vi "Set 2D Field (Polar)_mb.vi"(5 "error in":T2, 6 "f (radians)":dbl min=0.0 format="%.3f", 8 "Z-Axis Communications Config":T1={"GPIB address"=22, "GPIB bus"=0, "connection ID"=refnum, "IP"="192.168.2.200", "Active Comm Interface"=0, "Serial Port"="", "Programmer Type"=0} {"Programmer Type" items=["Model 430", "Model 420"]; "Active Comm Interface" items=["TCP/IP (Model 430 Only)", "RS232", "IEEE488"]}, 9 "Magnitude Limit (kG)":dbl format="%.3f", 10 "Y-Axis Communications Config":T1={"GPIB address"=22, "GPIB bus"=0, "connection ID"=refnum, "IP"="192.168.2.200", "Active Comm Interface"=0, "Serial Port"="", "Programmer Type"=0} {"Programmer Type" items=["Model 430", "Model 420"]; "Active Comm Interface" items=["TCP/IP (Model 430 Only)", "RS232", "IEEE488"]}, 11 "Field Magnitude r (kG)":dbl min=0.0 format="%.3f") -> (0 "Z-Axis Field (kG) out":dbl format="%.3f", 1 "Y-Axis Field (kG)":dbl format="%.3f", 3 "Within Limits?":bool, 4 "error out":T2)   [LabVIEW 2009]
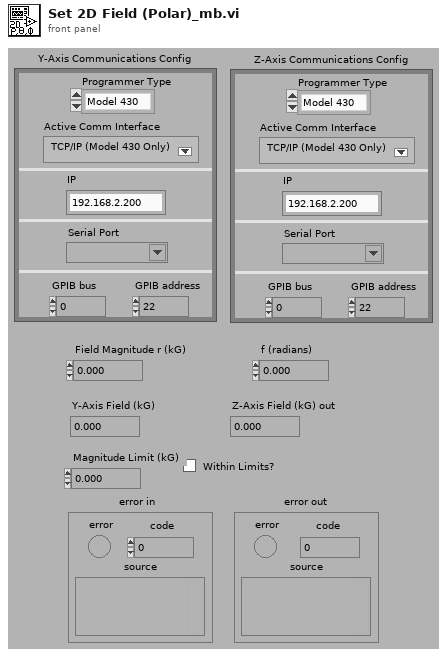
[diagram p1: front panel]
types:
  T1 = cluster{"GPIB address":i16, "GPIB bus":i16, "connection ID":refnum<k5>, "IP":string, "Active Comm Interface":u16, "Serial Port":refnum<visa-resource-name>, "Programmer Type":u16}
  T2 = cluster{"error":bool, "code":i32, "source":string}
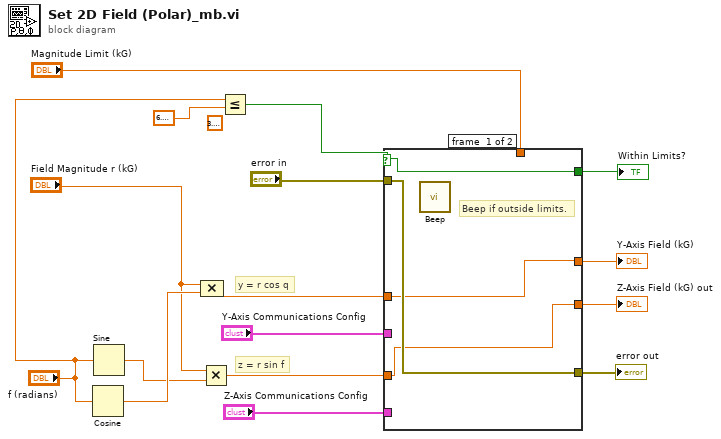
[diagram p0: block diagram]
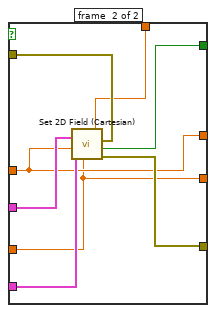
[diagram p2: hidden frame]
diagram:
  (unwired) 3.141592653589793
  # "z = r sin f"
  # "y = r cos q"
  n1 = Cosine(x="f (radians)") -> (cos(x)=w14:dbl)
  n2 = Sine(x="f (radians)") -> (sin(x)=w12:dbl)
  n3 = Compound Arithmetic op=MULTIPLY("Field Magnitude r (kG)", w14) -> (w13:dbl)
  n4 = Multiply(x="Field Magnitude r (kG)", y=w12) -> (x*y=w11:dbl)
  n5 = Less Or Equal?(x="f (radians)", y=6.283185307179586) -> (x <= y?=w6:bool)
  n6 = case shown="True" w6 {
    selector: w6 -> [w17 _]
    tunnel: "Y-Axis Communications Config" -> [_ w27]
    tunnel: w13 -> [w19 w23]
    tunnel: w11 -> [w18 w22]
    tunnel: "Z-Axis Communications Config" -> [_ w26]
    tunnel: "error in" -> [w20 w28]
    tunnel: [w20 w25] -> w15
    tunnel: [w17 w24] -> w10
    tunnel: [w19 w23] -> w9
    tunnel: [w18 w22] -> w8
    tunnel: "Magnitude Limit (kG)" -> [_ w21]
    frame #0 {
      # "Beep if outside limits."
      n7 = call <vilib>:"Beep.vi"() -> ()  [unwired: 12 in]
    }
    frame #1 {
      n8 = call <userlib>:"Set 2D Field (Cartesian).vi"("error in"=w28, "Magnitude Limit (kG)"=w21, "Z-Axis Field (kG)"=w22, "Z-Axis Communications Config"=w26, "Y-Axis Field (kG)"=w23, "Y-Axis Communications Config"=w27) -> ("error out"=w25:T2, "Within Limits?"=w24:bool)  [unwired: 2 in]
    }
  }
  "error out" <- w15
  "Y-Axis Field (kG)" <- w9
  "Z-Axis Field (kG) out" <- w8
  "Within Limits?" <- w10
